vi "Get Parent Actor Starting Folder Path.vi"(8 "error in (no error)":errorcluster) -> (0 "error out":errorcluster, 3 "Path String":path)   [LabVIEW 2020, in "Add Actor.lvlib"]
uses:
  Add Actor.lvlib
  <resource>/dialog/lvconfig.llb/LV Config Read Pathlist.vi
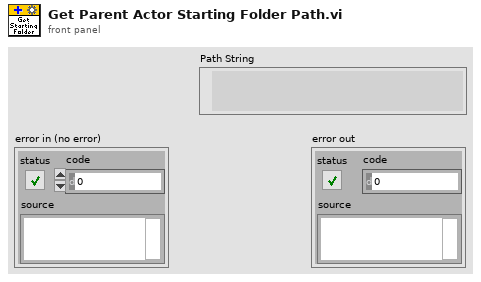
[diagram p1: front panel]
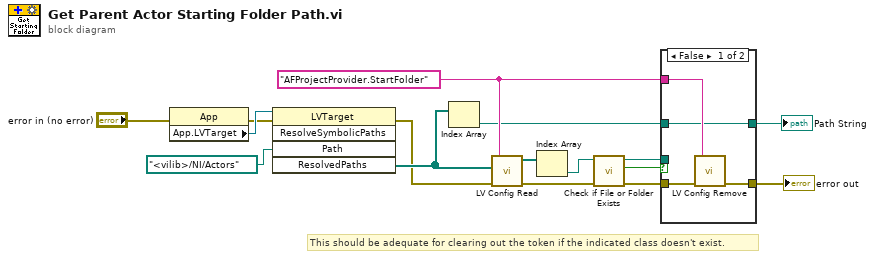
[diagram p0: block diagram]
diagram:
  w11 = "AFProjectProvider.StartFolder" ("key")
  # "This should be adequate for clearing out the token if the indicated class doesn't exist."
  n1 = property class="App"(error in="error in (no error)") -> (error out=w2:errorcluster, "App.LVTarget"=w7:refnum<vi>)  [unwired: 1 in, 1 out]
  n2 = invoke class="LVTarget" method="ResolveSymbolicPaths"(reference=w7, error in=w2, "Path"=path "<vilib>/NI/Actors") -> (error out=w3:errorcluster, "ResolvedPaths"=w5:path[])  [unwired: 2 in, 3 out]
  n3 = Index Array(array=w5) -> (element=w4:path)  [unwired: 1 in]
  n4 = call-poly <resource>:"LV Config Read.vi"("error in"=w3, "default value"=w5, "key"=w11) -> ("error out"=w14:errorcluster, "value"=w16:path[])  [unwired: 2 in, 1 out]
  n5 = Index Array(array=w16) -> (element=w15:path)  [unwired: 1 in]
  n6 = call <vilib>:"Check if File or Folder Exists.vi"("error in (no error)"=w14, "path"=w15) -> ("error out"=w13:errorcluster, "file or folder exists?"=w10:bool, "dup path"=w8:path)  [unwired: 7 in]
  n7 = case shown="False" w10 {
    tunnel: w13 -> [w20 w22]
    tunnel: [w19 w22] -> w12
    tunnel: w11 -> [w18 _]
    tunnel: w4 -> [w17 _]
    tunnel: [w17 w21] -> w9
    tunnel: w8 -> [_ w21]
    frame False {
      n8 = call <resource>:"LV Config Remove.vi"("error in"=w20, "key"=w18) -> ("error out"=w19:errorcluster)  [unwired: 5 in]
    }
    frame True {
    }
  }
  "error out" <- w12
  "Path String" <- w9
